vi "Test SplashWindow3.vi"   [LabVIEW 2020]
uses:
  a3eb0aa5-2cc5-4148-8f17-44e3bf90e6b5.vi
  a3eb0aa5-2cc5-4148-8f17-44e3bf90e6b5.vi/1b47866c-8e2d-43a7-815f-8cf18635e5a1.vi
  <userlib>/_NEVSTOP/TagDB/_Support/Change Detector/TagDB dbChanged.vi
  <userlib>/_NEVSTOP/TagDB/_Support/Error/_Clear Errors.vi
  a3eb0aa5-2cc5-4148-8f17-44e3bf90e6b5.vi/1b47866c-8e2d-43a7-815f-8cf18635e5a1.vi/29b2ea6d-6d7f-4e4a-ad31-a5cb760462c7.vi
  <userlib>/_NEVSTOP/TagDB/API/TagDB-Status.vi
  <userlib>/_NEVSTOP/TagDB/_Support/Change Detector/TagDB ChangeFlag.vi
  <userlib>/_NEVSTOP/TagDB/_Support/DataAccess/_NameCacher.vi
  <userlib>/_NEVSTOP/TagDB/_Support/Error/_[error50002]Invalid DataType.vi
  <userlib>/_NEVSTOP/TagDB/_Support/Error/_[error50000]Invalid DB REF.vi
  <userlib>/_NEVSTOP/TagDB/_Support/DataAccess/TagDB Ref to DVR.vi
  <userlib>/_NEVSTOP/TagDB/_Support/URL/TRIM-BOTH-SPACE.vi
  <userlib>/_NEVSTOP/TagDB/_Support/Error/_Build Error Cluster.vi
  <userlib>/_NEVSTOP/Communicable State Machine(CSM)/Communicable State Machine.lvlib
  <userlib>/_NEVSTOP/TagDB/Add-ons/RefManager/TagDB RefManager.lvlib
  <userlib>/_NEVSTOP/TagDB/TagDB.lvlib
  CSM-SplashWindow.lvlib
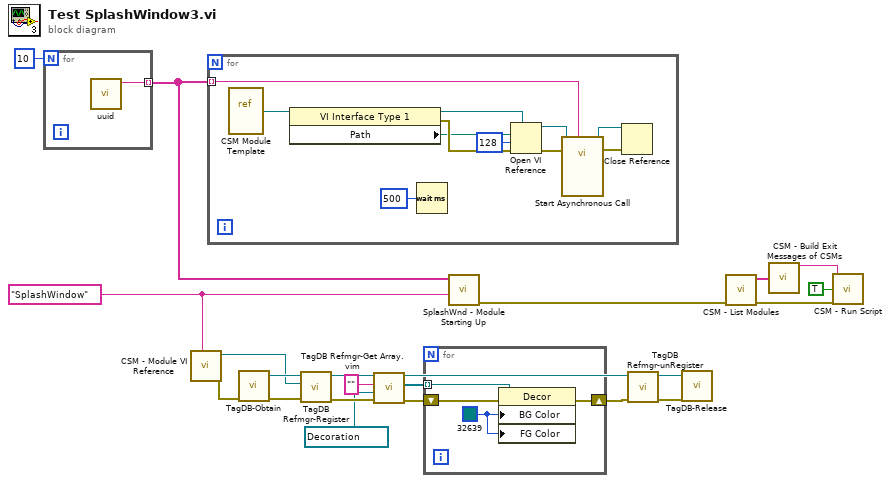
[diagram p0: block diagram]
diagram:
  w3 = "SplashWindow" ("Name (\"\" to Use UUID)")
  n1 = for {
    N: 10 -> [_]
    tunnel: [w23] -> w2 mode=indexing
    n2 = call <userlib>:"uuid.vi"() -> ("UUID"=w23:string)  [unwired: 11 in]
  }
  n3 = call <userlib>:"CSM - Module VI Reference.vi"("CSM Name"=w3) -> ("error out"=w9:errorcluster, "CSM Module VIRef"=w21:refnum<vi>)  [unwired: 9 in]
  n4 = for {
    tunnel: w2 -> [w24] mode=indexing
    n5 = vi-ref <userlib>:"CSM Module Template.vi"() -> (w27:refnum<vi>)
    n6 = property class="VI Interface Type 1"(reference=w27) -> (reference out=w31:refnum<vi>, error out=w29:errorcluster, "Path"=w28:path)  [unwired: 1 in]
    n7 = Wait (ms)(milliseconds to wait=u32 500) -> ()  [unwired: 1 out]
    n8 = Open VI Reference(type specifier VI Refnum (for type only)=w31, vi path=w28, options=128, error in (no error)=w29) -> (vi reference=w30:refnum<vi>, error out=w26:errorcluster)  [unwired: 2 in]
    n9 = call-by-ref "Start Asynchronous Call"(reference=w30, error in=w26, "Name (\"\" to Use UUID)"=w24) -> (reference out=w33:refnum<vi>, error out=w32:errorcluster)  [unwired: 11 in]
    n10 = Close Reference(reference=w33, error in (no error)=w32) -> ()  [unwired: 1 out]
  }
  n11 = call <userlib>:"TagDB-Obtain.vi"("error in (no error)"=w9) -> ("error out"=w20:errorcluster, "TagDB"=w22:refnum<k1>)  [unwired: 4 in, 1 out]
  n12 = call <userlib>:"TagDB Refmgr-Register.vi"("error in (no error)"=w20, "VI Refnum"=w21, "TagDB in"=w22) -> ("error out"=w18:errorcluster, "TagDB out"=w19:refnum<k1>)  [unwired: 6 in, 1 out]
  n13 = call "TagDB Refmgr-Get Array.vim"("error in (no error)"=w18, "Type"=refnum<vi> refnum, "RegExp"="", "DB Ref"=w19) -> ("error out"=w13:errorcluster, "References"=w11:refnum<vi>[], "DB Ref(dup)"=w12:refnum<k1>)  [unwired: 4 in, 1 out]
  n14 = for {
    shift-right: [w37] -> w14
    shift-left: w13 -> [w38]
    tunnel: w11 -> [w36] mode=indexing
    w35 = u32 32639 ("Colors:BG Color")
    n15 = property class="Decor"(reference=w36, error in=w38, "BG Color"=w35, "FG Color"=w35) -> (error out=w37:errorcluster)  [unwired: 1 out]
  }
  n16 = call "SplashWnd - Module Starting Up.vi"("Name (\"\" to Use UUID)"=w3, "Modules"=w2) -> ("error out"=w1:errorcluster)  [unwired: 9 in]
  n17 = call <userlib>:"TagDB Refmgr-unRegister.vi"("error in (no error)"=w14, "TagDB in"=w12) -> ("error out"=w16:errorcluster, "TagDB out"=w15:refnum<k1>)  [unwired: 8 in]
  n18 = call <userlib>:"TagDB-Release.vi"("error in (no error)"=w16, "TagDB"=w15) -> ()  [unwired: 9 in, 1 out]
  n19 = call <userlib>:"CSM - List Modules.vi"("Error In"=w1) -> ("error out"=w5:errorcluster, "Module Names"=w8:string[])  [unwired: 9 in]
  n20 = call <userlib>:"CSM - Build Exit Messages of CSMs.vi"("CSMs"=w8) -> ("States"=w7:string)  [unwired: 14 in]
  n21 = call <userlib>:"CSM - Run Script.vi"("CSM Scripts"=w7, "Continue If Error? (F)"=TRUE, "error in (no error)"=w5) -> ()  [unwired: 10 in, 3 out]
